vi "XYZ Stage Loop.vi"(6 "Used functions":bool, 8 "error in":errorcluster, 9 "Configuration":T1={"Parameter Analizer"={"Parameter Analyzer VISA Session"="COM1", "Sweeping Time Parameters"={"Integration Time"=0, "Short Integration Time (s)"=1.0, "Long Integration Time (s)"=0.0, "Wait Time Parameter"=1.0}, "Acquisition Mode"=enum."Sweeping Mode", "Status Polling Time (ms)"=0, "Comment"="Test VI", "SMU 1 - Sweeping"={"Start / Offset"=0.0, "Stop / Ratio"=1.0, "Step \n(linear only)"=0.01, "Compliance"=0.1, "Power \nCompliance"=0.0, "Mode"=0, "Function"=0, "Sweep Mode"=FALSE}, "SMU 2 - Sweeping"={"Start / Offset"=0.0, "Stop / Ratio"=1.0, "Step \n(linear only)"=0.01, "Compliance"=0.1, "Power \nCompliance"=0.0, "Mode"=0, "Function"=0, "Sweep Mode"=FALSE}, "SMU 3 - Sweeping"={"Start / Offset"=0.0, "Stop / Ratio"=1.0, "Step \n(linear only)"=0.01, "Compliance"=0.1, "Power \nCompliance"=0.0, "Mode"=0, "Function"=0, "Sweep Mode"=FALSE}, "SMU 4 - Sweeping"={"Start / Offset"=0.0, "Stop / Ratio"=1.0, "Step \n(linear only)"=0.01, "Compliance"=0.1, "Power \nCompliance"=0.0, "Mode"=0, "Function"=0, "Sweep Mode"=FALSE}, "Sweep Spacing"=0, "Range"=0, "SMU1 - Sampling"={"Source"=10.0, "Compliance"=1e-05, "Mode"=0, "Function"=FALSE}, "SMU2 - Sampling"={"Source"=1.0, "Compliance"=1.0, "Mode"=0, "Function"=FALSE}, "SMU3 - Sampling"={"Source"=10.0, "Compliance"=1e-05, "Mode"=0, "Function"=FALSE}, "SMU4 - Sampling"={"Source"=0.1, "Compliance"=60.0, "Mode"=10, "Function"=FALSE}, "Sampling Time Parameters"={"Initial Interval (s)"=0.1, "Number of Samples"=60, "Total Sampling Time (s)"=10.0, "Hold Time (s)"=0.0, "Sampling Mode"=0, "Sampling Time"=0}, "Stop Condition"={"Enable Delay (s)"=0.0, "Name"="", "Threshold"=0.0, "num. of events"=1, "Event"=0, "Stop Condition Enable"=FALSE}}, "Switching Matrix"={"Switching Matrix VISA Session"="GPIB0::18::INSTR", "Connections"=[{"Connections"=[FALSE, FALSE, FALSE, FALSE, FALSE, FALSE, FALSE, FALSE, FALSE, FALSE, FALSE, FALSE], "Connection Type"=enum."Disconnected"}, {"Connections"=[FALSE, FALSE, FALSE, FALSE, FALSE, FALSE, FALSE, FALSE, FALSE, FALSE, FALSE, FALSE], "Connection Type"=enum."Disconnected"}, {"Connections"=[FALSE, FALSE, FALSE, FALSE, FALSE, FALSE, FALSE, FALSE, FALSE, FALSE, FALSE, FALSE], "Connection Type"=enum."Disconnected"}, {"Connections"=[FALSE, FALSE, FALSE, FALSE, FALSE, FALSE, FALSE, FALSE, FALSE, FALSE, FALSE, FALSE], "Connection Type"=enum."Disconnected"}, {"Connections"=[FALSE, FALSE, FALSE, FALSE, FALSE, FALSE, FALSE, FALSE, FALSE, FALSE, FALSE, FALSE], "Connection Type"=enum."Disconnected"}, {"Connections"=[FALSE, FALSE, FALSE, FALSE, FALSE, FALSE, FALSE, FALSE, FALSE, FALSE, FALSE, FALSE], "Connection Type"=enum."Disconnected"}, {"Connections"=[FALSE, FALSE, FALSE, FALSE, FALSE, FALSE, FALSE, FALSE, FALSE, FALSE, FALSE, FALSE], "Connection Type"=enum."Disconnected"}, {"Connections"=[FALSE, FALSE, FALSE, FALSE, FALSE, FALSE, FALSE, FALSE, FALSE, FALSE, FALSE, FALSE], "Connection Type"=enum."Disconnected"}]}, "Stress Control"={"Stress Control VISA Session"="StrainMotor", "Axis"=0, "Motion"=0, "Destination (°)"=0.0, "Speed (°/s)"=4.0, "Position (°)"=25.0}, "Optical Spectrometer"={"Laser Settings"={"Laser Wavelength"=enum."365 nm", "Neutral Density Filter"=enum."100%"}, "Spectrometer Settings"={"Confocal Hole Size (µm)"=0.0, "Grating"=2, "Detector"=enum."InGaAs Array"}, "Acquisition Settings"={"Acquisition Mode"=enum."Multi-Window", "Spectal Position (nm)"=632.0, "From (nm)"=735.0, "To (nm)"=0.0, "Integration Time (s)"=0.0, "Number of Accumulations"=3, "AutoScanning"=FALSE, "Spike Removal"=FALSE}, "Path"=path "C:/07 - Prizes and Awards/Marie Curie Prize/Reply Editors Final NCOMMS(10).docx"}, "Switches & Mirrors"={"Relay VISA Session"="COM1", "Switches"={"Laser"=FALSE, "Video"=FALSE}, "Delays (ms)"={"Laser"=500, "Video"=1500}}, "Camera"={"Settings"={"Pixel clock"=20, "Frame rate"=30.0, "Exposure time"=33.21525, "Master Gain"=0, "Red Gain"=0, "Green Gain"=0, "Blue Gain"=0, "Auto Gain"=FALSE, "White-balance"=FALSE, "Color Correction"=FALSE}}, "XYZ Stage"={"Connection Settings"={"Tango VISA"="", "Baudrate"=57600, "Show Protocol?"=FALSE}, "Manual Control"={"North"=FALSE, "South"=FALSE, "West"=FALSE, "East"=FALSE, "Up"=FALSE, "Down"=FALSE, "Stop"=FALSE, "XY Step"=0.0, "Z step"=0.0}, "Coordinate Control"={"Motion Mode"=enum."Absolute", "Destination [mm]"=[]}}, "AutoFocus"={"Matching Criteria"={"Minimum Score"=700.0, "Color Score Weight"=700.0, "Minimum Contrast"=50, "Match Mode"=0, "Match Feature Mode"=0, "Subpixel Accuracy"=TRUE, "Color Sensitivity"=1, "Search Strategy"=1}, "Z Scan Parameters"={"Z Range"=1380.0, "Resolution"=5000.0, "Initial Direction"=enum."Up", "Focus Threshold"=0.1, "Ascent Constant"=0.1}, "Displacement"=0.0, "Transformation Matrix"=[]}, "Sava Data"={"Workspace Info"={"Device Name"="ProberHead_Tst_C29K3_7(2)", "Device Info"="ProberHead_Tst_C29", "Path"=path "C:/Users/gio/Desktop/ProbeHeadTest"}, "Instrument Configuration"={"Instrument"=enum."Unknown Instrument", "Configuration"="Test Configuration"}, "Stress Motor Position"=0.0, "Electrical Measurement"={"Sequence"=[], "V1"=[], "V2"=[], "V3"=[], "V4"=[], "I1"=[], "I2"=[], "I3"=[], "I4"=[]}, "Optical Spectrum"={"Intensity"=[], "Wavelength"=[], "Energy"=[], "Raman Shift"=[], "Detector Temperature"=0.0}}, "PlotData"={"Sliders"={"Strain Sequence"=0, "Instrument Sequence"=0}, "Measurement"={"Which Instrument?"=enum."No Plot", "Electrical Measurement"={"Sequence"=[], "V1"=[], "V2"=[], "V3"=[], "V4"=[], "I1"=[], "I2"=[], "I3"=[], "I4"=[]}, "Measurement Mode"=enum."Sweeping Mode", "Optical Spectrum"={"Intensity"=[], "Wavelength"=[], "Energy"=[], "Raman Shift"=[], "Detector Temperature"=0.0}}, "Instrument Steps"=[], "Strain Points"=[]}, "Instrument Sequence"={"Caller VI"=enum."User"}, "Strain Measurement"={"Stress Sequence "={"Max Motor Position"=1380.0, "# Intermediate Points"=5000, "Initial Direction"=enum."Tension"}, "Track?"=FALSE}} {"AutoFocus"."Displacement" scale=1.0..1000.0; "AutoFocus"."Z Scan Parameters"."Focus Threshold" min=0.0 max=1000.0 step=1.0 format="%#_2f"; "AutoFocus"."Z Scan Parameters"."Ascent Constant" min=0.0 max=1000.0 step=1.0 format="%#_2f"; "AutoFocus"."Z Scan Parameters"."Resolution" min=0.0 max=1.0 step=0.01 format="%_2g"; "AutoFocus"."Z Scan Parameters"."Z Range" format="%_3g"; "AutoFocus"."Matching Criteria"."Match Mode" items=["Shift Invariant", "Rotation Invariant"]; "AutoFocus"."Matching Criteria"."Match Feature Mode" items=["Color and Shape", "Color", "Shape"]; "AutoFocus"."Matching Criteria"."Color Sensitivity" items=["Low Sensitivity", "Medium Sensitivity", "High Sensitivity"]; "AutoFocus"."Matching Criteria"."Search Strategy" items=["Conservative", "Balance", "Aggressive", "Very Aggressive"]; "XYZ Stage"."Manual Control"."Z step" scale=0.1..10.0; "XYZ Stage"."Manual Control"."XY Step" scale=0.1..1000.0; "Camera"."Settings"."Blue Gain" min=0 max=100 scale=0.0..100.0; "Camera"."Settings"."Green Gain" min=0 max=100 scale=0.0..100.0; "Camera"."Settings"."Red Gain" min=0 max=100 scale=0.0..100.0; "Camera"."Settings"."Master Gain" min=0 max=100 scale=0.0..100.0; "Camera"."Settings"."Exposure time" min=0.101625 max=159.246375 step=0.101625 scale=0.101625..159.246375 scale format="%#.3g"; "Camera"."Settings"."Frame rate" min=2.7455631699174137 max=6.2675785993528725 step=0.000101625 scale=2.7455631699174137..6.2675785993528725 scale format="%^#_3g"; "Camera"."Settings"."Pixel clock" min=5 max=43 scale=5.0..43.0; "PlotData"."Sliders"."Instrument Sequence" scale=0.0..10.0; "PlotData"."Sliders"."Strain Sequence" scale=0.0..10.0; "Strain Measurement"."Stress Sequence"."# Intermediate Points" max=1390; "Parameter Analizer"."Stop Condition"."Event" items=["Value > Threshold", "Value < Threshold", "| Value | > | Threshold |", "| Value | < | Threshold |"]; "Parameter Analizer"."Stop Condition"."Threshold" format="%^.2e"; "Parameter Analizer"."Stop Condition"."Enable Delay (s)" format="%.1f"; "Parameter Analizer"."Sampling Time Parameters"."Sampling Time" items=["Auto (linear only)", "No Limit", "Set Limit"]; "Parameter Analizer"."Sampling Time Parameters"."Sampling Mode" items=["Linear", "Log10", "Log25", "Log50", "Thinned Out"]; "Parameter Analizer"."Sampling Time Parameters"."Hold Time (s)" format="%.4f"; "Parameter Analizer"."Sampling Time Parameters"."Total Sampling Time (s)" format="%.1f"; "Parameter Analizer"."Sampling Time Parameters"."Initial Interval (s)" format="%^.3e"; "Parameter Analizer"."SMU 4 - Sweeping"."Function" items=["Disabled", "Var 1", "Var 2", "Var 1'", "Constant"]; "Parameter Analizer"."SMU 4 - Sweeping"."Mode" items=["V", "I", "V pulse", "I  pulse", "Common"]; "Parameter Analizer"."SMU 4 - Sweeping"."Power \nCompliance" format="%^.2e"; "Parameter Analizer"."SMU 4 - Sweeping"."Compliance" format="%^.2e"; "Parameter Analizer"."SMU 4 - Sweeping"."Step \n(linear only)" format="%^.4e"; "Parameter Analizer"."SMU 4 - Sweeping"."Stop / Ratio" format="%^.4e"; "Parameter Analizer"."SMU 4 - Sweeping"."Start / Offset" format="%^.4e"; "Parameter Analizer"."SMU 3 - Sweeping"."Function" items=["Disabled", "Var 1", "Var 2", "Var 1'", "Constant"]; "Parameter Analizer"."SMU 3 - Sweeping"."Mode" items=["V", "I", "V pulse", "I  pulse", "Common"]; "Parameter Analizer"."SMU 3 - Sweeping"."Power \nCompliance" format="%^.2e"; "Parameter Analizer"."SMU 3 - Sweeping"."Compliance" format="%^.2e"; "Parameter Analizer"."SMU 3 - Sweeping"."Step \n(linear only)" format="%^.4e"; "Parameter Analizer"."SMU 3 - Sweeping"."Stop / Ratio" format="%^.4e"; "Parameter Analizer"."SMU 3 - Sweeping"."Start / Offset" format="%^.4e"; "Parameter Analizer"."SMU 2 - Sweeping"."Function" items=["Disabled", "Var 1", "Var 2", "Var 1'", "Constant"]; "Parameter Analizer"."SMU 2 - Sweeping"."Mode" items=["V", "I", "V pulse", "I  pulse", "Common"]; "Parameter Analizer"."SMU 2 - Sweeping"."Power \nCompliance" format="%^.2e"; "Parameter Analizer"."SMU 2 - Sweeping"."Compliance" format="%^.2e"; "Parameter Analizer"."SMU 2 - Sweeping"."Step \n(linear only)" format="%^.4e"; "Parameter Analizer"."SMU 2 - Sweeping"."Stop / Ratio" format="%^.4e"; "Parameter Analizer"."SMU 2 - Sweeping"."Start / Offset" format="%^.4e"; "Parameter Analizer"."SMU 1 - Sweeping"."Function" items=["Disabled", "Var 1", "Var 2", "Var 1'", "Constant"]; "Parameter Analizer"."SMU 1 - Sweeping"."Mode" items=["V", "I", "V pulse", "I  pulse", "Common"]; "Parameter Analizer"."SMU 1 - Sweeping"."Power \nCompliance" format="%^.2e"; "Parameter Analizer"."SMU 1 - Sweeping"."Compliance" format="%^.2e"; "Parameter Analizer"."SMU 1 - Sweeping"."Step \n(linear only)" format="%^.4e"; "Parameter Analizer"."SMU 1 - Sweeping"."Stop / Ratio" format="%^.4e"; "Parameter Analizer"."SMU 1 - Sweeping"."Start / Offset" format="%^.4e"; "Parameter Analizer"."Sweeping Time Parameters"."Long Integration Time (s)" scale=0.02..2.0; "Parameter Analizer"."Sweeping Time Parameters"."Short Integration Time (s)" scale=8e-05..0.00192; "Parameter Analizer"."Sweeping Time Parameters"."Integration Time" items=["Short", "Long"]; "Parameter Analizer"."Sweeping Time Parameters"."Wait Time Parameter" format="%.1f"; "Parameter Analizer"."SMU4 - Sampling"."Mode" items=["V", "I", "Common"]; "Parameter Analizer"."SMU4 - Sampling"."Compliance" format="%^.2e"; "Parameter Analizer"."SMU4 - Sampling"."Source" format="%^.3e"; "Parameter Analizer"."SMU3 - Sampling"."Mode" items=["V", "I", "Common"]; "Parameter Analizer"."SMU3 - Sampling"."Compliance" format="%^.2e"; "Parameter Analizer"."SMU3 - Sampling"."Source" format="%^.3e"; "Parameter Analizer"."SMU2 - Sampling"."Mode" items=["V", "I", "Common"]; "Parameter Analizer"."SMU2 - Sampling"."Compliance" format="%^.2e"; "Parameter Analizer"."SMU2 - Sampling"."Source" format="%^.3e"; "Parameter Analizer"."SMU1 - Sampling"."Mode" items=["V", "I", "Common"]; "Parameter Analizer"."SMU1 - Sampling"."Compliance" format="%^.2e"; "Parameter Analizer"."SMU1 - Sampling"."Source" format="%^.3e"; "Parameter Analizer"."Range" items=["auto", "fixed", "limited"]; "Parameter Analizer"."Sweep Spacing" items=["linear", "log 10", "log 25", "log 50"]; "Stress Control"."Axis" min=1 max=3; "Stress Control"."Position (°)" format="%.6g"; "Stress Control"."Speed (°/s)" min=0.0 max=4.0 format="%.6f"; "Stress Control"."Destination (°)" min=-2000000000.0 max=2000000000.0 format="%.6f"; "Stress Control"."Motion" items=["Absolute", "Relative"]; "Optical Spectrometer"."Spectrometer Settings"."Grating" items=["1800 l/mm", "150 l/mm"]}, 10 "Message Queues out":T57, 11 "Notifiers":T44) -> (0 "error out":errorcluster)   [LabVIEW 2014]
uses:
  support/Message Queue/All Message Queues.ctl
  support/Message Queue/Message Cluster.ctl
  support/Notifiers/Notifiers.ctl
  support/Message Handler Loop Notifiers.ctl
  Hardware Control/Parameter Analyzer/Parameter Analyzer Notifiers.ctl
  Hardware Control/Switching Matrix/Switching Matrix Notifiers.ctl
  Hardware Control/Stress Control/StressControl Notifiers.ctl
  Hardware Control/Spectrometer/Spectrometer Notifiers.ctl
  Hardware Control/Switches and Mirrors/SwitchesMirrors Notifiers.ctl
  Hardware Control/Camera/Camera Notifiers.ctl
  Hardware Control/XYZ Stage/XYZ Notifications.ctl
  Hardware Control/Autofocus/Autofocus Notifiers.ctl
  Measurements/Optoelectronic Measurement/Optoelectronic Notifiers.ctl
  Measurements/Save Data/SaveData Notifiers.ctl
  Measurements/Instrument Sequence/Instrument Sequence Notifiers.ctl
  support/Configuration/Configuration.ctl
  Hardware Control/Parameter Analyzer/Parameter Analyzer Config.ctl
  Hardware Control/Parameter Analyzer/Parameter Analyzer Integration Parameters.ctl
  Hardware Control/Parameter Analyzer/Parameter Analyzer SMU Sweeping.ctl
  Hardware Control/Parameter Analyzer/Parameter Analyzer Sweep Spacing.ctl
  Hardware Control/Parameter Analyzer/Parameter Analyzer SMU Range.ctl
  Hardware Control/Parameter Analyzer/Parameter Analyzer SMU Sampling.ctl
  Hardware Control/Parameter Analyzer/Parameter Analyzer Sampling Parameters.ctl
  Hardware Control/Parameter Analyzer/Parameter Analyzer Stop Sampling Conditions.ctl
  Hardware Control/Switching Matrix/Switching Matrix Config.ctl
  Hardware Control/Stress Control/StressControl Config.ctl
  Hardware Control/Spectrometer/Spectrometer Config.ctl
  Hardware Control/Spectrometer/Laser Settings.ctl
  Hardware Control/Spectrometer/Laser.ctl
  Hardware Control/Spectrometer/Filter.ctl
  Hardware Control/Spectrometer/Grating Detector Settings.ctl
  Hardware Control/Spectrometer/Grating.ctl
  Hardware Control/Spectrometer/Detector.ctl
  Hardware Control/Spectrometer/Acquisition Settings.ctl
  Hardware Control/Switches and Mirrors/SwitchesMirrors Config.ctl
  Hardware Control/Switches and Mirrors/SwitchesMirrors Status.ctl
  Hardware Control/Camera/Camera Config.ctl
  Hardware Control/Camera/Camera Settings.ctl
  Hardware Control/XYZ Stage/XYZ Config.ctl
  Hardware Control/XYZ Stage/XYZ Connection Settings.ctl
  Hardware Control/XYZ Stage/XYZ Stage Control.ctl
  Hardware Control/XYZ Stage/XYZ Coordinate Control.ctl
  Hardware Control/Autofocus/AutoFocus Config.ctl
  Hardware Control/Autofocus/ZScan.ctl
  <vilib>/Analysis/Matrix/Datatypes/RealMatrix.ctl
  Measurements/Save Data/SaveData Config.ctl
  Measurements/Save Data/SaveData Workspace Info.ctl
  Measurements/Save Data/SaveData Instrument Configuration.ctl
  Measurements/Instrument Sequence/Instrument List.ctl
  Hardware Control/Spectrometer/Spectral Data.ctl
  Measurements/Plot Data/PlotData Config.ctl
  Measurements/Plot Data/Measurement.ctl
  Measurements/Plot Data/WhichInstrument.ctl
  Hardware Control/Parameter Analyzer/Electrical Data.ctl
  Measurements/Instrument Sequence/Instrument Steps.ctl
  Measurements/Instrument Sequence/Action.ctl
  Measurements/Instrument Sequence/Instrument Sequence Config.ctl
  Measurements/Strain Measurement/Strain Measurement Config.ctl
  Hardware Control/XYZ Stage/XYZ Function.ctl
  support/Message Queue/Message Queue.lvlib
  <vilib>/Analysis/Matrix/NI_Matrix.lvlib
panel:
  # "LICENSED MATERIALS – PROPERTY OF IBM\nCopyright IBM Corp. 2016,\nALL RIGHTS RESERVED"
  # "XY"
  # "Z"
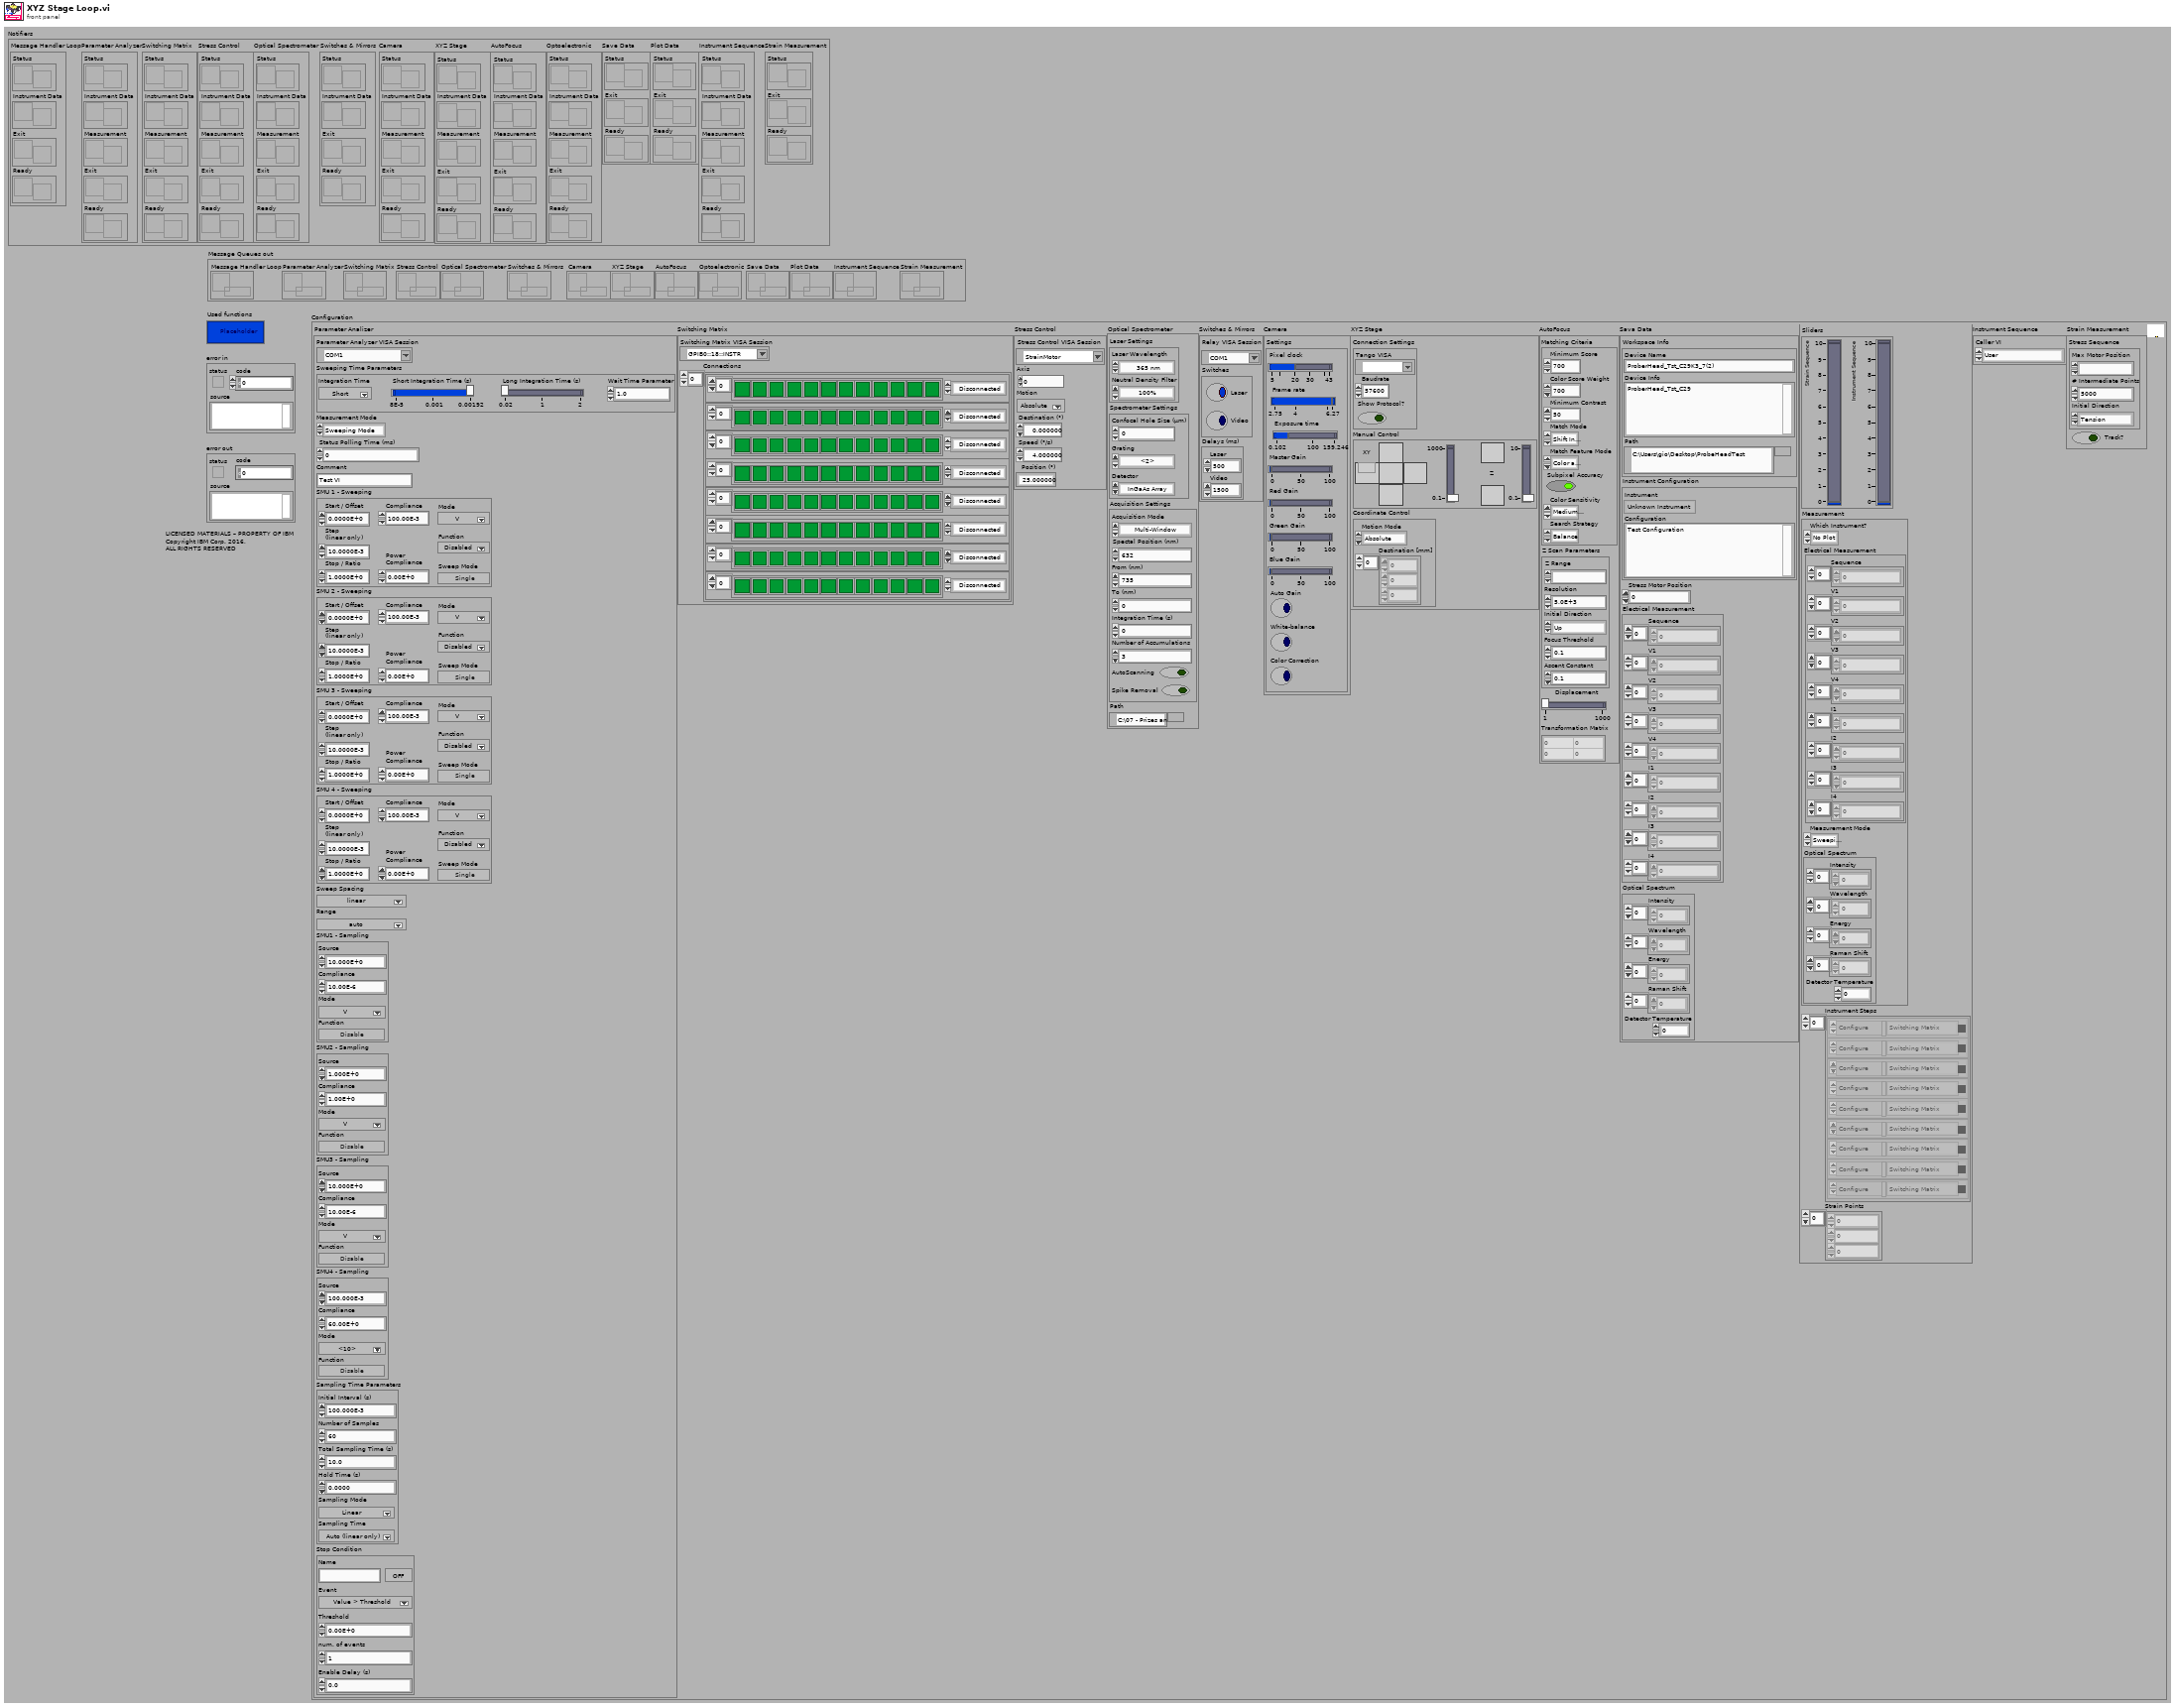
[diagram p1: front panel]
types:
  T1 = typedef "Configuration.ctl" = cluster{"Parameter Analizer":T2, "Switching Matrix":T10, "Stress Control":T11, "Optical Spectrometer":T12, "Switches & Mirrors":T20, "Camera":T22, "XYZ Stage":T24, "AutoFocus":T28, "Sava Data":T31, "PlotData":T36, "Instrument Sequence":T42, "Strain Measurement":T43}
  T2 = typedef "Parameter Analyzer Config.ctl" = cluster{"Parameter Analyzer VISA Session":refnum<visa-resource-name>, "Sweeping Time Parameters":T3, "Acquisition Mode":enum32{"Sweeping Mode", "Sampling Mode"}, "Status Polling Time (ms)":u32, "Comment":string, "SMU 1 - Sweeping":T4, "SMU 2 - Sweeping":T4, "SMU 3 - Sweeping":T4, "SMU 4 - Sweeping":T4, "Sweep Spacing":T5, "Range":T6, "SMU1 - Sampling":T7, "SMU2 - Sampling":T7, "SMU3 - Sampling":T7, "SMU4 - Sampling":T7, "Sampling Time Parameters":T8, "Stop Condition":T9}
  T3 = typedef "Parameter Analyzer Integration Parameters.ctl" = cluster{"Integration Time":u32, "Short Integration Time (s)":dbl, "Long Integration Time (s)":dbl, "Wait Time Parameter":dbl}
  T4 = typedef "Parameter Analyzer SMU Sweeping.ctl" = cluster{"Start / Offset":dbl, "Stop / Ratio":dbl, "Step \n(linear only)":dbl, "Compliance":dbl, "Power \nCompliance":dbl, "Mode":u32, "Function":i32, "Sweep Mode":bool}
  T5 = typedef "Parameter Analyzer Sweep Spacing.ctl" = u16
  T6 = typedef "Parameter Analyzer SMU Range.ctl" = u16
  T7 = typedef "Parameter Analyzer SMU Sampling.ctl" = cluster{"Source":dbl, "Compliance":dbl, "Mode":u32, "Function":bool}
  T8 = typedef "Parameter Analyzer Sampling Parameters.ctl" = cluster{"Initial Interval (s)":dbl, "Number of Samples":i32, "Total Sampling Time (s)":dbl, "Hold Time (s)":dbl, "Sampling Mode":i32, "Sampling Time":i32}
  T9 = typedef "Parameter Analyzer Stop Sampling Conditions.ctl" = cluster{"Enable Delay (s)":dbl, "Name":string, "Threshold":dbl, "num. of events":i32, "Event":i32, "Stop Condition Enable":bool}
  T10 = typedef "Switching Matrix Config.ctl" = cluster{"Switching Matrix VISA Session":refnum<visa-resource-name>, "Connections":cluster{"Connections":bool[], "Connection Type":enum16{"Disconnected", "Make - Break", "Break - Make"}}[]}
  T11 = typedef "StressControl Config.ctl" = cluster{"Stress Control VISA Session":refnum<visa-resource-name>, "Axis":i32, "Motion":u16, "Destination (°)":dbl, "Speed (°/s)":dbl, "Position (°)":dbl}
  T12 = typedef "Spectrometer Config.ctl" = cluster{"Laser Settings":T13, "Spectrometer Settings":T16, "Acquisition Settings":T19, "Path":path}
  T13 = typedef "Laser Settings.ctl" = cluster{"Laser Wavelength":T14, "Neutral Density Filter":T15}
  T14 = typedef "Laser.ctl" = enum16{"633 nm", "784 nm", "532 nm", "365 nm"}
  T15 = typedef "Filter.ctl" = enum16{"100%", "50%", "25%", "10%", "1%", "0.1%", "0.01%"}
  T16 = typedef "Grating Detector Settings.ctl" = cluster{"Confocal Hole Size (µm)":dbl, "Grating":T17, "Detector":T18}
  T17 = typedef "Grating.ctl" = u16
  T18 = typedef "Detector.ctl" = enum16{"InGaAs Array", "Silicon CCD"}
  T19 = typedef "Acquisition Settings.ctl" = cluster{"Acquisition Mode":enum16{"Single Window", "Multi-Window"}, "Spectal Position (nm)":dbl, "From (nm)":dbl, "To (nm)":dbl, "Integration Time (s)":dbl, "Number of Accumulations":i32, "AutoScanning":bool, "Spike Removal":bool}
  T20 = typedef "SwitchesMirrors Config.ctl" = cluster{"Relay VISA Session":refnum<visa-resource-name>, "Switches":T21, "Delays (ms)":cluster{"Laser":u32, "Video":u32}}
  T21 = typedef "SwitchesMirrors Status.ctl" = cluster{"Laser":bool, "Video":bool}
  T22 = typedef "Camera Config.ctl" = cluster{"Settings":T23}
  T23 = typedef "Camera Settings.ctl" = cluster{"Pixel clock":i32, "Frame rate":dbl, "Exposure time":dbl, "Master Gain":i32, "Red Gain":i32, "Green Gain":i32, "Blue Gain":i32, "Auto Gain":bool, "White-balance":bool, "Color Correction":bool}
  T24 = typedef "XYZ Config.ctl" = cluster{"Connection Settings":T25, "Manual Control":T26, "Coordinate Control":T27}
  T25 = typedef "XYZ Connection Settings.ctl" = cluster{"Tango VISA":refnum<visa-resource-name>, "Baudrate":i32, "Show Protocol?":bool}
  T26 = typedef "XYZ Stage Control.ctl" = cluster{"North":bool, "South":bool, "West":bool, "East":bool, "Up":bool, "Down":bool, "Stop":bool, "XY Step":dbl, "Z step":dbl}
  T27 = typedef "XYZ Coordinate Control.ctl" = cluster{"Motion Mode":enum16{"Absolute", "Relative"}, "Destination [mm]":dbl[]}
  T28 = typedef "AutoFocus Config.ctl" = cluster{"Matching Criteria":cluster{"Minimum Score":sgl, "Color Score Weight":sgl, "Minimum Contrast":i32, "Match Mode":u32, "Match Feature Mode":u32, "Subpixel Accuracy":bool, "Color Sensitivity":u32, "Search Strategy":u32}, "Z Scan Parameters":T29, "Displacement":dbl, "Transformation Matrix":T30}
  T29 = typedef "ZScan.ctl" = cluster{"Z Range":ext, "Resolution":dbl, "Initial Direction":enum16{"Up", "Down"}, "Focus Threshold":dbl, "Ascent Constant":dbl}
  T30 = typedef "NI_Matrix.lvlib/RealMatrix.ctl" = dbl[][]
  T31 = typedef "SaveData Config.ctl" = cluster{"Workspace Info":T32, "Instrument Configuration":T33, "Stress Motor Position":dbl, "Electrical Measurement":cluster{"Sequence":dbl[], "V1":dbl[], "V2":dbl[], "V3":dbl[], "V4":dbl[], "I1":dbl[], "I2":dbl[], "I3":dbl[], "I4":dbl[]}, "Optical Spectrum":T35}
  T32 = typedef "SaveData Workspace Info.ctl" = cluster{"Device Name":string, "Device Info":string, "Path":path}
  T33 = typedef "SaveData Instrument Configuration.ctl" = cluster{"Instrument":T34, "Configuration":string}
  T34 = typedef "Instrument List.ctl" = enum32{"Unknown Instrument", "Switching Matrix", "Parameter Analyzer", "Optical Spectrometer", "Optoelectronic", "Autofocus"}
  T35 = typedef "Spectral Data.ctl" = cluster{"Intensity":dbl[], "Wavelength":dbl[], "Energy":dbl[], "Raman Shift":dbl[], "Detector Temperature":dbl}
  T36 = typedef "PlotData Config.ctl" = cluster{"Sliders":cluster{"Strain Sequence":i32, "Instrument Sequence":i32}, "Measurement":T37, "Instrument Steps":T40, "Strain Points":dbl[]}
  T37 = typedef "Measurement.ctl" = cluster{"Which Instrument?":T38, "Electrical Measurement":T39, "Measurement Mode":enum16{"Sweeping Mode", "Sampling Mode"}, "Optical Spectrum":T35}
  T38 = typedef "WhichInstrument.ctl" = enum16{"No Plot", "Spectrometer", "Parameter Analyzer", "Optoelectronic"}
  T39 = typedef "Electrical Data.ctl" = cluster{"Sequence":dbl[], "V1":dbl[], "V2":dbl[], "V3":dbl[], "V4":dbl[], "I1":dbl[], "I2":dbl[], "I3":dbl[], "I4":dbl[]}
  T40 = typedef "Instrument Steps.ctl" = cluster{"Action":T41, "Configuration":variant, "Instrument":T34, "Status":enum8{"False", "True", "Mixed"}}[]
  T41 = typedef "Action.ctl" = enum32{"Configure", "Measure"}
  T42 = typedef "Instrument Sequence Config.ctl" = cluster{"Caller VI":enum16{"User", "Stress Measurement VI"}}
  T43 = typedef "Strain Measurement Config.ctl" = cluster{"Stress Sequence ":cluster{"Max Motor Position":ext, "# Intermediate Points":u32, "Initial Direction":enum16{"Tension", "Compression"}}, "Track?":bool}
  T44 = typedef "Notifiers.ctl" = cluster{"Message Handler Loop":T45, "Parameter Analyzer":T46, "Switching Matrix":T47, "Stress Control":T48, "Optical Spectrometer":T49, "Switches & Mirrors":T50, "Camera":T51, "XYZ Stage":T52, "AutoFocus":T53, "Optoelectronic":T54, "Save Data":T55, "Plot Data":T55, "Instrument Sequence":T56, "Strain Measurement":cluster{"Status":refnum<notifier>, "Exit":refnum<notifier>, "Ready":refnum<notifier>}}
  T45 = typedef "Message Handler Loop Notifiers.ctl" = cluster{"Status":refnum<notifier>, "Instrument Data":refnum<notifier>, "Exit":refnum<notifier>, "Ready":refnum<notifier>}
  T46 = typedef "Parameter Analyzer Notifiers.ctl" = cluster{"Status":refnum<notifier>, "Instrument Data":refnum<notifier>, "Measurement":refnum<notifier>, "Exit":refnum<notifier>, "Ready":refnum<notifier>}
  T47 = typedef "Switching Matrix Notifiers.ctl" = cluster{"Status":refnum<notifier>, "Instrument Data":refnum<notifier>, "Measurement":refnum<notifier>, "Exit":refnum<notifier>, "Ready":refnum<notifier>}
  T48 = typedef "StressControl Notifiers.ctl" = cluster{"Status":refnum<notifier>, "Instrument Data":refnum<notifier>, "Measurement":refnum<notifier>, "Exit":refnum<notifier>, "Ready":refnum<notifier>}
  T49 = typedef "Spectrometer Notifiers.ctl" = cluster{"Status":refnum<notifier>, "Instrument Data":refnum<notifier>, "Measurement":refnum<notifier>, "Exit":refnum<notifier>, "Ready":refnum<notifier>}
  T50 = typedef "SwitchesMirrors Notifiers.ctl" = cluster{"Status":refnum<notifier>, "Instrument Data":refnum<notifier>, "Exit":refnum<notifier>, "Ready":refnum<notifier>}
  T51 = typedef "Camera Notifiers.ctl" = cluster{"Status":refnum<notifier>, "Instrument Data":refnum<notifier>, "Measurement":refnum<notifier>, "Exit":refnum<notifier>, "Ready":refnum<notifier>}
  T52 = typedef "XYZ Notifications.ctl" = cluster{"Status":refnum<notifier>, "Instrument Data":refnum<notifier>, "Measurement":refnum<notifier>, "Exit":refnum<notifier>, "Ready":refnum<notifier>}
  T53 = typedef "Autofocus Notifiers.ctl" = cluster{"Status":refnum<notifier>, "Instrument Data":refnum<notifier>, "Measurement":refnum<notifier>, "Exit":refnum<notifier>, "Ready":refnum<notifier>}
  T54 = typedef "Optoelectronic Notifiers.ctl" = cluster{"Status":refnum<notifier>, "Instrument Data":refnum<notifier>, "Measurement":refnum<notifier>, "Exit":refnum<notifier>, "Ready":refnum<notifier>}
  T55 = typedef "SaveData Notifiers.ctl" = cluster{"Status":refnum<notifier>, "Exit":refnum<notifier>, "Ready":refnum<notifier>}
  T56 = typedef "Instrument Sequence Notifiers.ctl" = cluster{"Status":refnum<notifier>, "Instrument Data":refnum<notifier>, "Measurement":refnum<notifier>, "Exit":refnum<notifier>, "Ready":refnum<notifier>}
  T57 = typedef "Message Queue.lvlib/All Message Queues.ctl" = cluster{"Message Handler Loop":refnum<queue>, "Parameter Analyzer":refnum<queue>, "Switching Matrix":refnum<queue>, "Stress Control":refnum<queue>, "Optical Spectrometer":refnum<queue>, "Switches & Mirrors":refnum<queue>, "Camera":refnum<queue>, "XYZ Stage":refnum<queue>, "AutoFocus":refnum<queue>, "Optoelectronic":refnum<queue>, "Save Data":refnum<queue>, "Plot Data":refnum<queue>, "Instrument Sequence":refnum<queue>, "Strain Measurement":refnum<queue>}
  T58 = typedef "XYZ Data.ctl" = cluster{"Configuration":T24, "Refnums":T59, "Initialization":T60}
  T59 = typedef "XYZ Refnums.ctl" = cluster{"Instrument Status":refnum<vi>, "Position":refnum<vi>, "Manual Control":refnum<vi>, "Up":refnum<vi>, "Down":refnum<vi>, "North":refnum<vi>, "South":refnum<vi>, "East":refnum<vi>, "West":refnum<vi>, "Stop":refnum<vi>, "Limits":refnum<vi>}
  T60 = typedef "XYZ Initialization.ctl" = cluster{"Update Visa Session":bool, "Set To Default":bool, "Get Status":bool, "Update Refnums":bool}
  T61 = typedef "XYZ Function.ctl" = enum16{"Connect", "Initialize", "Calibrate", "Meaure Range", "Limits", "Center", "Set Zero", "Velocity", "Manual Control", "Coordinate Move", "Move with Backlash Compensation", "Meander", "Sequence", "Analog Output", "Send Command", "Show Protocol", "Get Status", "Disconnect", "Update Refnums"}
  T62 = cluster{"Connected?":bool, "LSID":i32, "Position":dbl[], "Number of Axes":u8}
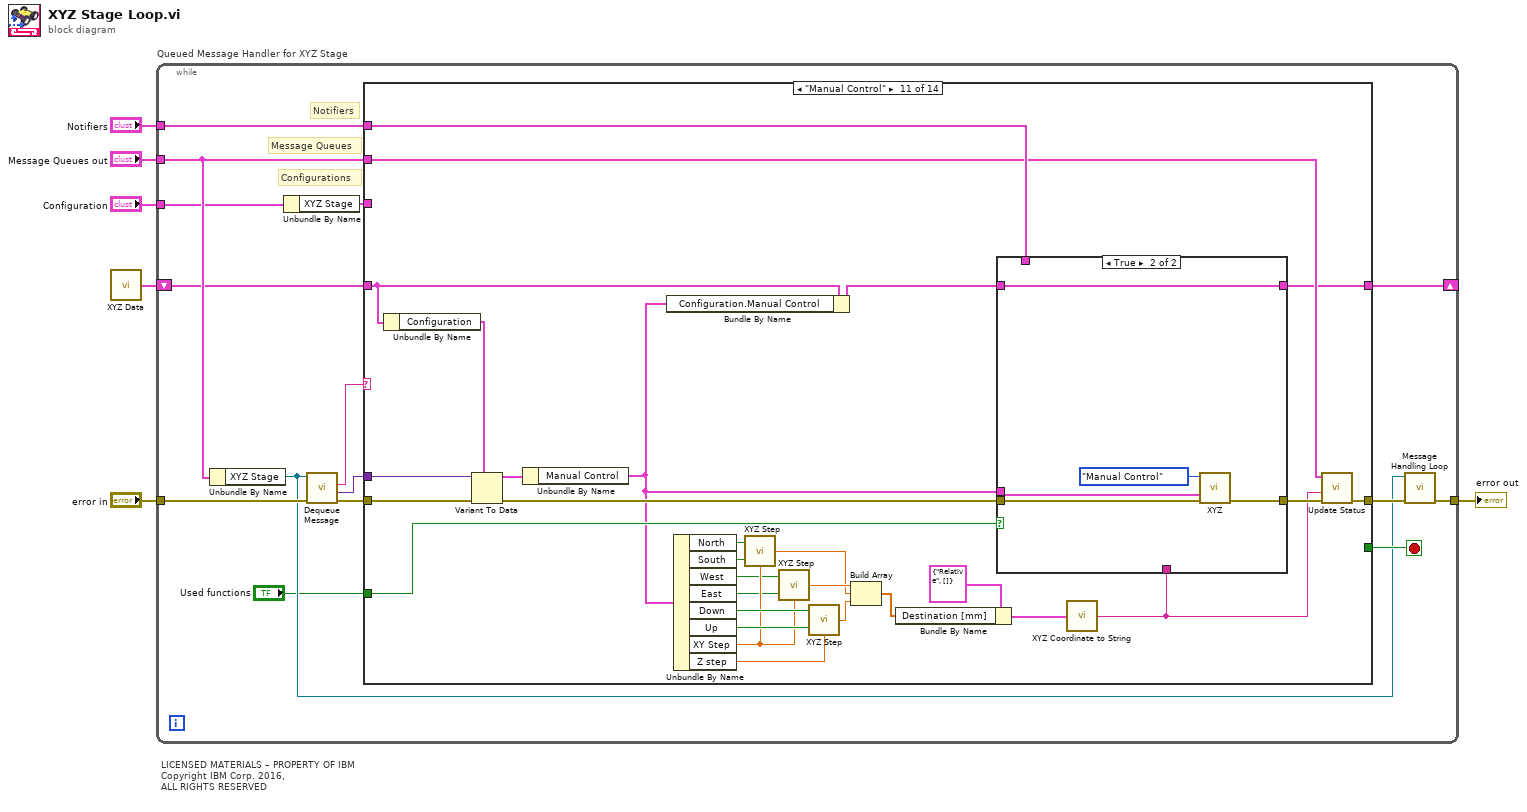
[diagram p0: block diagram]
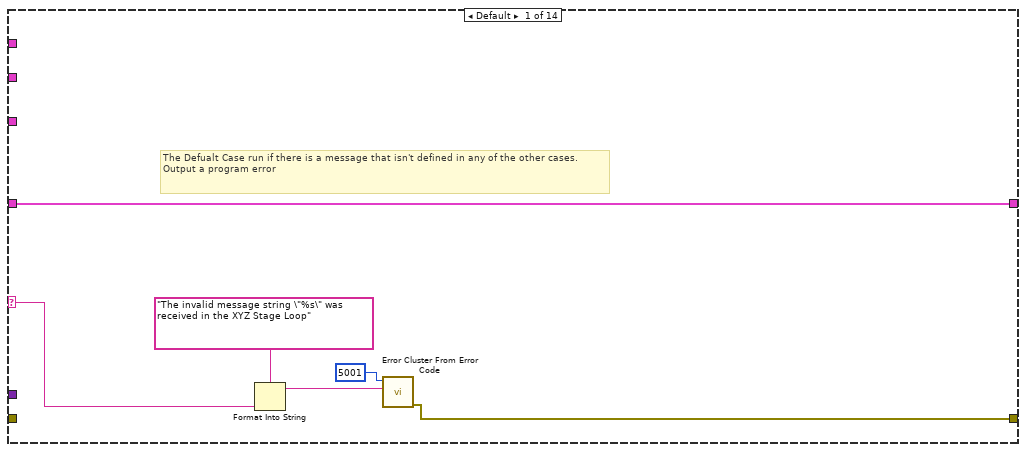
[diagram p2: hidden frame]
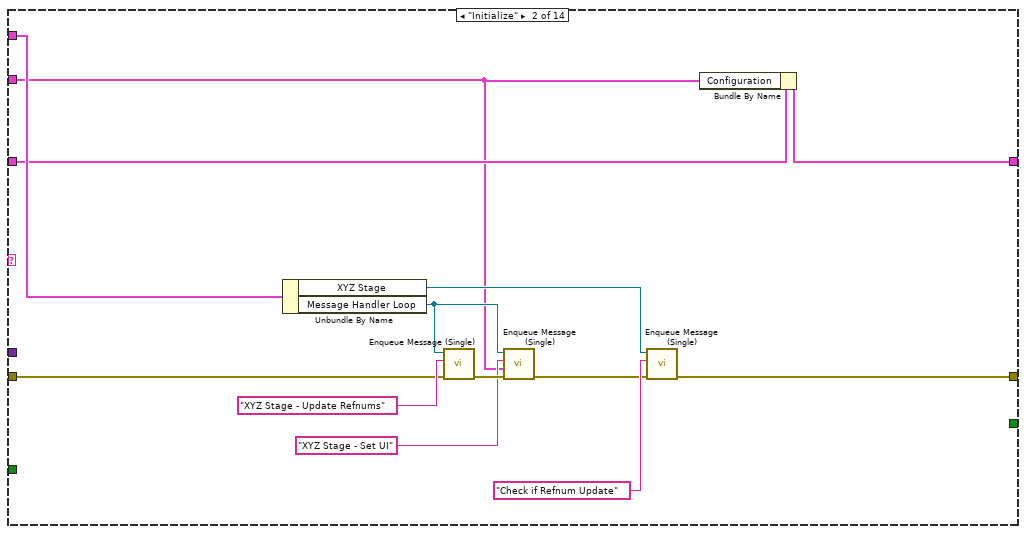
[diagram p3: hidden frame]
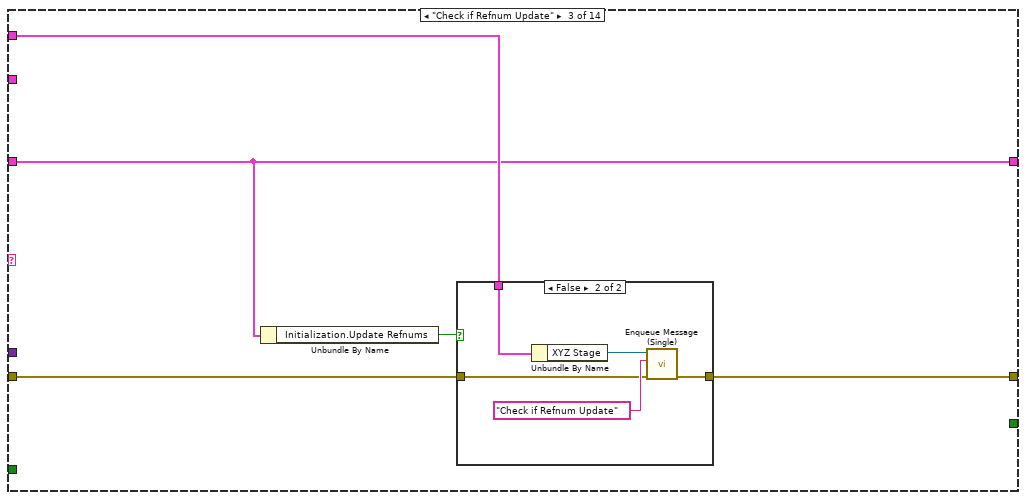
[diagram p4: hidden frame]
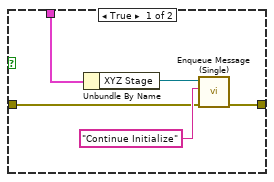
[diagram p5: hidden frame]
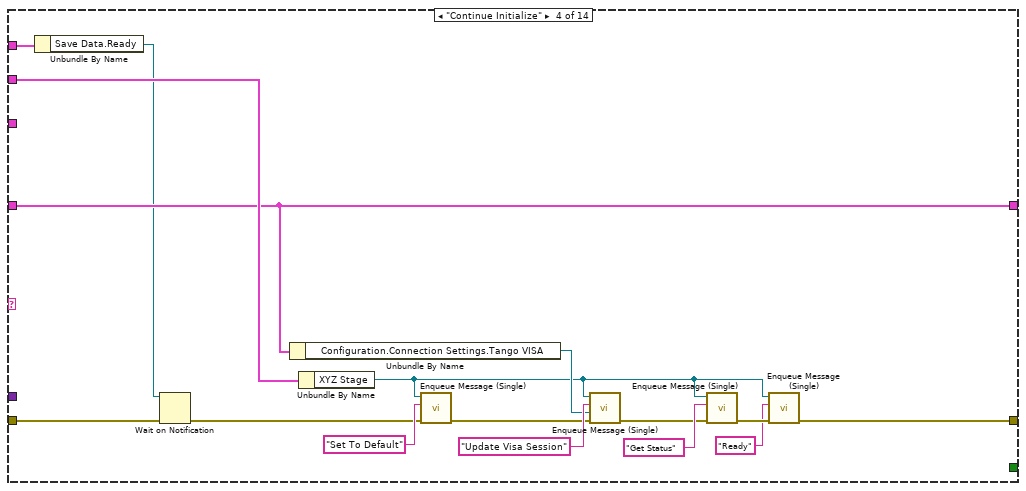
[diagram p6: hidden frame]
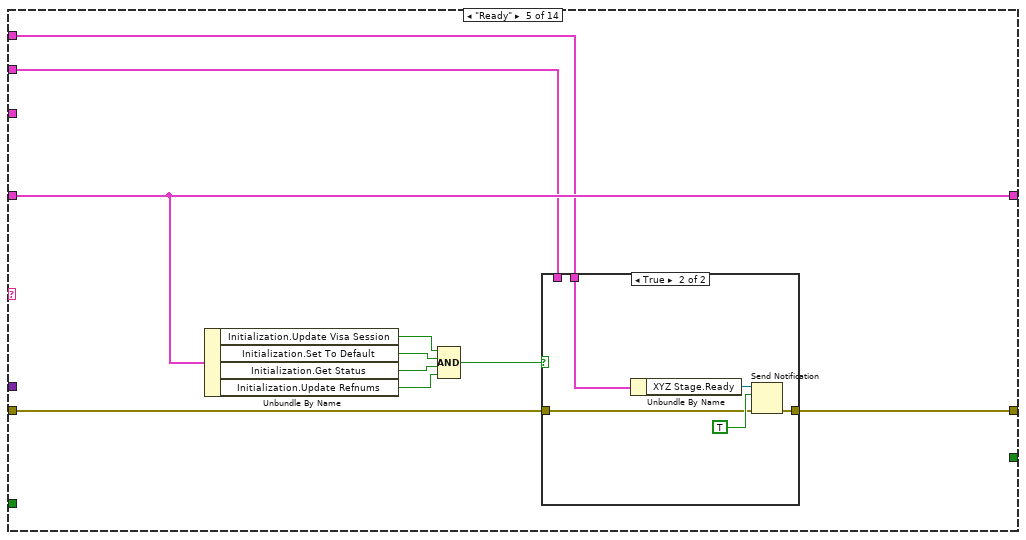
[diagram p7: hidden frame]
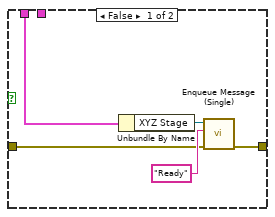
[diagram p8: hidden frame]
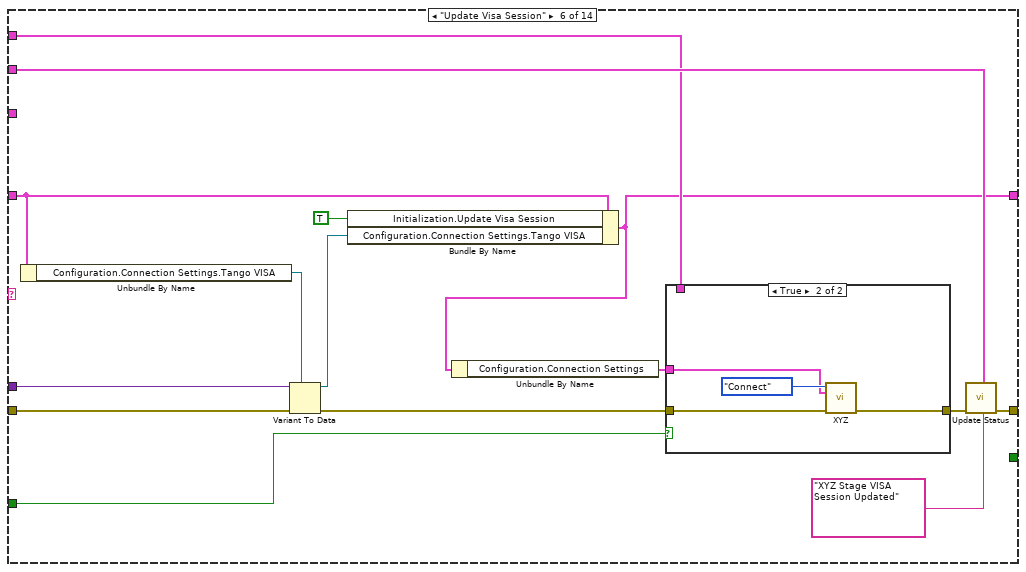
[diagram p9: hidden frame]
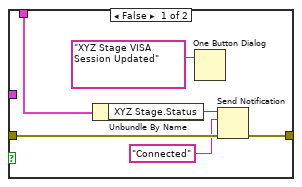
[diagram p10: hidden frame]
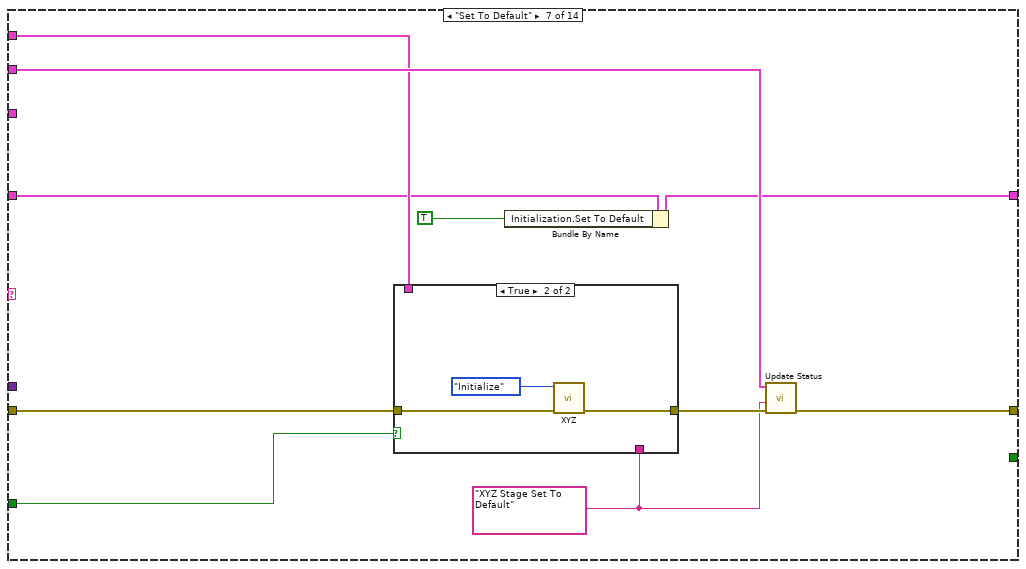
[diagram p11: hidden frame]
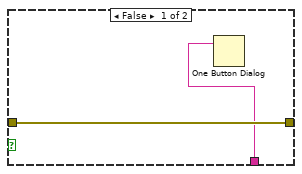
[diagram p12: hidden frame]
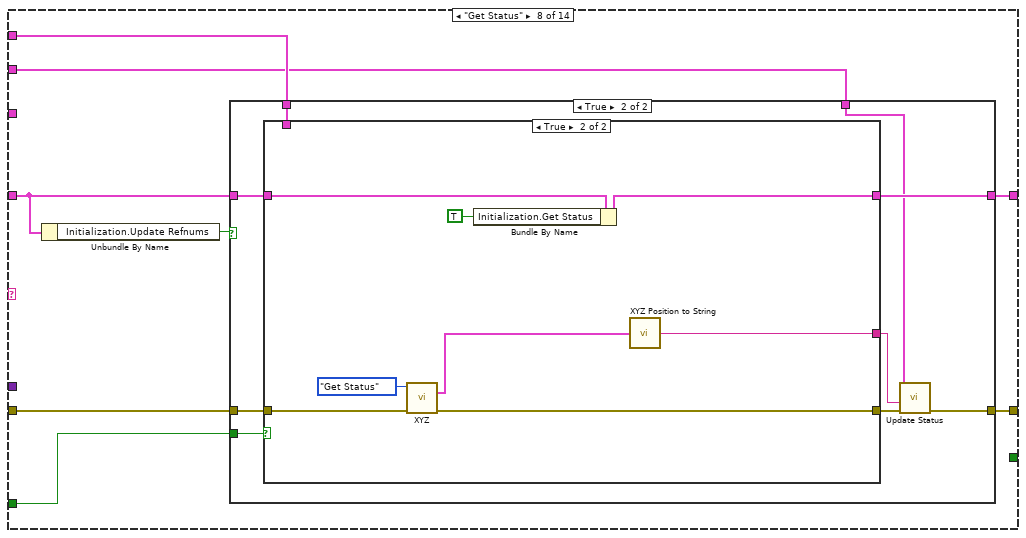
[diagram p13: hidden frame]
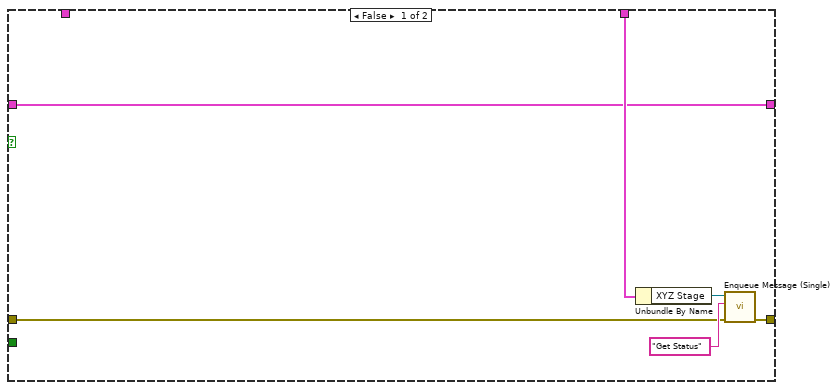
[diagram p14: hidden frame]
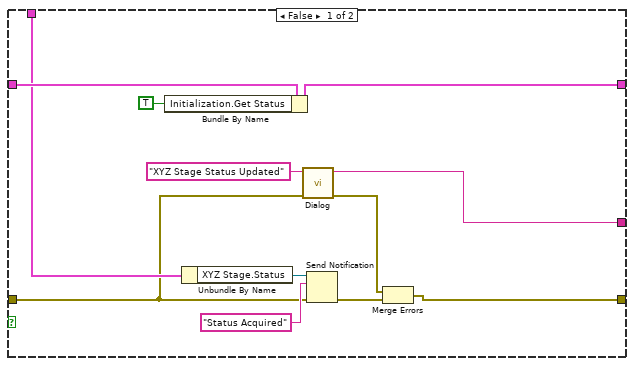
[diagram p15: hidden frame]
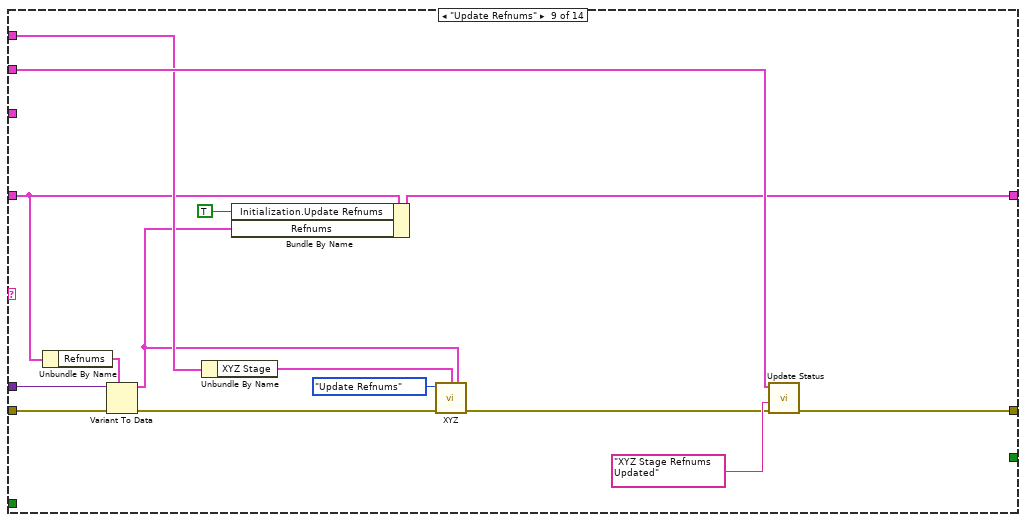
[diagram p16: hidden frame]
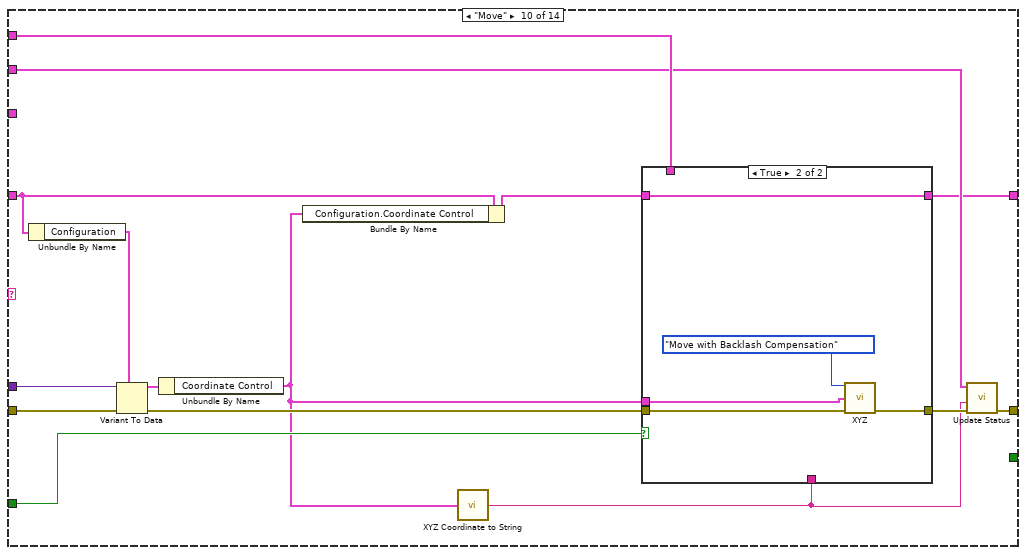
[diagram p17: hidden frame]
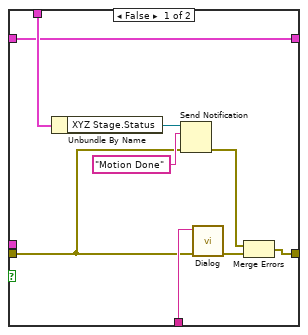
[diagram p18: hidden frame]
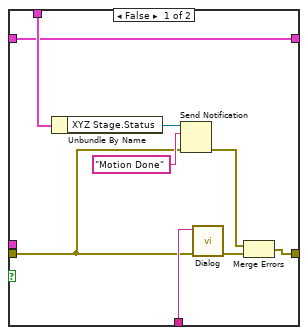
[diagram p19: hidden frame]
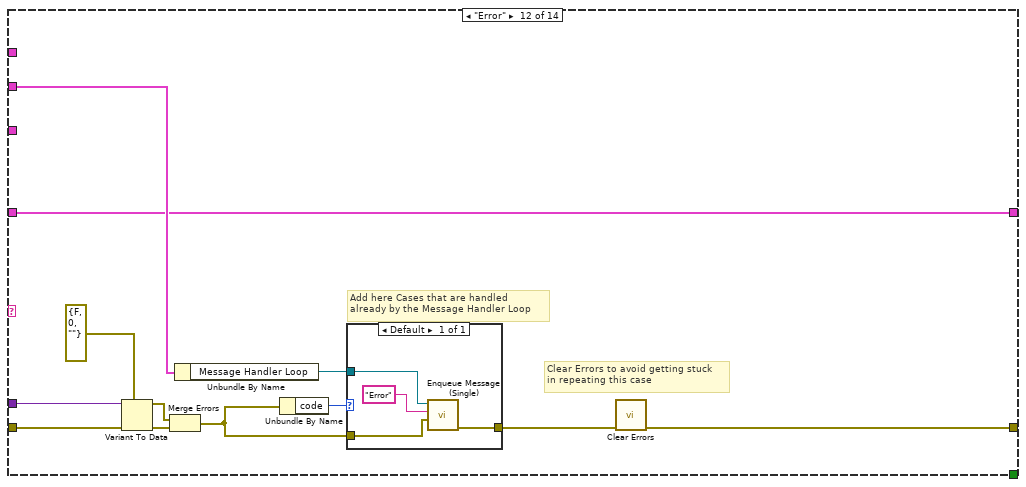
[diagram p20: hidden frame]
diagram:
  # "LICENSED MATERIALS – PROPERTY OF IBM\nCopyright IBM Corp. 2016,\nALL RIGHTS RESERVED"
  n1 = call "XYZ Data.vi"() -> ("XYZ Stage Data"=w1:T58)
  n2 = while "Queued Message Handler for XYZ Stage" {
    tunnel: "error in" -> [w21]
    tunnel: [w13] -> w2
    tunnel: "Message Queues out" -> [w17]
    tunnel: "Notifiers" -> [w16]
    tunnel: "Configuration" -> [w11]
    shift-right: [w7] -> _
    shift-left: w1 -> [w8]
    stop <- w15 stop-if-true
    # "Configurations"
    # "Notifiers"
    # "Message Queues"
    n3 = Unbundle By Name(w17) -> ("XYZ Stage"=w12:refnum<queue>)
    n4 = Unbundle By Name(w11) -> ("XYZ Stage"=w10:T24)
    n5 = call "Dequeue Message.vi"("error in (no error)"=w21, "Message Queue"=w12) -> ("error out"=w20:errorcluster, "Message Data"=w18:variant, "Message"=w19:string)  [unwired: 7 out]
    n6 = case shown="\"Manual Control\"" w19 {
      selector: w19 -> [w24 _ _ _ _ _ _ _ _ _ _ _ _ _]
      tunnel: w20 -> [_ w28 w43 w57 w75 w104 w118 w134 w187 w201 w244 w269 w287 w303]
      tunnel: [w23 w29 w44 w68 w73 w102 w125 w132 w186 w199 w242 w264 w277 w302] -> w14
      tunnel: w18 -> [_ _ _ _ _ w106 _ _ w188 w203 w246 w262 _ _]
      tunnel: w17 -> [_ w40 w45 w71 w74 w101 w124 w135 w184 w195 w238 w270 w289 _]
      tunnel: w16 -> [_ _ _ w58 w72 w98 w122 w136 w183 w196 w239 _ w279 w301]
      tunnel: [_ _ _ _ _ _ _ _ _ _ _ _ TRUE ("Priority Message? (F)") _] -> w15
      tunnel: w10 -> [_ w31 _ _ _ _ _ _ _ _ _ _ _ _]
      tunnel: w8 -> [w22 w39 w42 w66 w79 w96 w119 w137 w180 w192 w235 w261 w284 w299]
      tunnel: "Used functions" -> [_ _ _ _ _ w103 w126 w139 _ w200 w243 _ w285 _]
      tunnel: [w22 w37 w42 w66 w79 w93 w121 w138 w182 w194 w237 w261 w284 w299] -> w7
      frame Default {
        # "The Defualt Case run if there is a message that isn't defined in any of the other cases.\nOutput a program error"
        n7 = Format Into String(format string="The invalid message string \"%s\" was  received in the XYZ Stage Loop", w24) -> (resulting string=w26:string)  [unwired: 2 in, 1 out]
        n8 = call <vilib>:"Error Cluster From Error Code.vi"("error message (\"\")"=w26, "error code (0)"=5001) -> ("error out"=w23:errorcluster)  [unwired: 2 in, 5 out]
      }
      frame "Initialize" {
        n9 = Unbundle By Name(w40) -> ("XYZ Stage"=w35:refnum<queue>, "Message Handler Loop"=w32:refnum<queue>)
        n10 = call "Enqueue Message (Single).vi"("error in (no error)"=w28, "Message"="XYZ Stage - Update Refnums", "Message Queue"=w32) -> ("error out"=w34:errorcluster)  [unwired: 1 in, 7 out]
        n11 = call "Enqueue Message (Single).vi"("error in (no error)"=w34, "Message Data"=w31, "Message"="XYZ Stage - Set UI", "Message Queue"=w32) -> ("error out"=w30:errorcluster)  [unwired: 7 out]
        n12 = call "Enqueue Message (Single).vi"("error in (no error)"=w30, "Message"="Check if Refnum Update", "Message Queue"=w35) -> ("error out"=w29:errorcluster)  [unwired: 1 in, 7 out]
        n13 = Bundle By Name(cluster=w39, "Configuration"=w31) -> (w37:T58)
      }
      frame "Check if Refnum Update" {
        n14 = Unbundle By Name(w42) -> ("Initialization.Update Refnums"=w41:bool)
        n15 = case shown="False" w41 {
          tunnel: w45 -> [w50 w55]
          tunnel: [w47 w52] -> w44
          tunnel: w43 -> [w46 w51]
          frame True {
            n16 = Unbundle By Name(w50) -> ("XYZ Stage"=w48:refnum<queue>)
            n17 = call "Enqueue Message (Single).vi"("error in (no error)"=w46, "Message"="Continue Initialize", "Message Queue"=w48) -> ("error out"=w47:errorcluster)  [unwired: 1 in, 7 out]
          }
          frame False {
            n18 = Unbundle By Name(w55) -> ("XYZ Stage"=w53:refnum<queue>)
            n19 = call "Enqueue Message (Single).vi"("error in (no error)"=w51, "Message"="Check if Refnum Update", "Message Queue"=w53) -> ("error out"=w52:errorcluster)  [unwired: 1 in, 7 out]
          }
        }
      }
      frame "Continue Initialize" {
        n20 = Unbundle By Name(w58) -> ("Save Data.Ready"=w59:refnum<notifier>)
        n21 = Wait on Notification(notifier=w59, error in (no error)=w57) -> (error out=w56:errorcluster)  [unwired: 2 in, 3 out]
        n22 = Unbundle By Name(w66) -> ("Configuration.Connection Settings.Tango VISA"=w65:refnum<visa-resource-name>)
        n23 = Unbundle By Name(w71) -> ("XYZ Stage"=w62:refnum<queue>)
        n24 = call "Enqueue Message (Single).vi"("error in (no error)"=w56, "Message"="Set To Default", "Message Queue"=w62) -> ("error out"=w63:errorcluster)  [unwired: 1 in, 7 out]
        n25 = call "Enqueue Message (Single).vi"("error in (no error)"=w63, "Message Data"=w65, "Message"="Update Visa Session", "Message Queue"=w62) -> ("error out"=w61:errorcluster)  [unwired: 7 out]
        n26 = call "Enqueue Message (Single).vi"("error in (no error)"=w61, "Message"="Get Status", "Message Queue"=w62) -> ("error out"=w69:errorcluster)  [unwired: 1 in, 7 out]
        n27 = call "Enqueue Message (Single).vi"("error in (no error)"=w69, "Message"="Ready", "Message Queue"=w62) -> ("error out"=w68:errorcluster)  [unwired: 1 in, 7 out]
      }
      frame "Ready" {
        n28 = Unbundle By Name(w79) -> ("Initialization.Update Visa Session"=w80:bool, "Initialization.Set To Default"=w76:bool, "Initialization.Get Status"=w77:bool, "Initialization.Update Refnums"=w78:bool)
        n29 = Compound Arithmetic op=AND(w80, w76, w77, w78) -> (w81:bool)
        n30 = case shown="True" w81 {
          tunnel: [w84 w89] -> w73
          tunnel: w75 -> [w83 w88]
          tunnel: w74 -> [w82 _]
          tunnel: w72 -> [_ w87]
          frame False {
            n31 = Unbundle By Name(w82) -> ("XYZ Stage"=w86:refnum<queue>)
            n32 = call "Enqueue Message (Single).vi"("error in (no error)"=w83, "Message"="Ready", "Message Queue"=w86) -> ("error out"=w84:errorcluster)  [unwired: 1 in, 7 out]
          }
          frame True {
            n33 = Unbundle By Name(w87) -> ("XYZ Stage.Ready"=w90:refnum<notifier>)
            n34 = Send Notification(notification=TRUE, notifier=w90, error in (no error)=w88) -> (error out=w89:errorcluster)  [unwired: 1 out]
          }
        }
      }
      frame "Update Visa Session" {
        n35 = Unbundle By Name(w96) -> ("Configuration.Connection Settings.Tango VISA"=w95:refnum<visa-resource-name>)
        n36 = Variant To Data(error in=w104, type=w95, Variant=w106) -> (data=w94:refnum<visa-resource-name>, error out=w105:errorcluster)
        n37 = Bundle By Name(cluster=w96, "Initialization.Update Visa Session"=TRUE, "Configuration.Connection Settings.Tango VISA"=w94) -> (w93:T58)
        n38 = Unbundle By Name(w93) -> ("Configuration.Connection Settings"=w92:T25)
        n39 = case shown="True" w103 {
          tunnel: w105 -> [w110 w115]
          tunnel: [w109 w113] -> w99
          tunnel: w98 -> [w112 _]
          tunnel: w92 -> [_ w114]
          frame False {
            n40 = Unbundle By Name(w112) -> ("XYZ Stage.Status"=w111:refnum<notifier>)
            n41 = One Button Dialog(message="XYZ Stage VISA Session Updated" ("button name (\"OK\")")) -> ()  [unwired: 2 out]
            n42 = Send Notification(notification="Connected", notifier=w111, error in (no error)=w110) -> (error out=w109:errorcluster)  [unwired: 1 out]
          }
          frame True {
            n43 = call "XYZ.vi"("Function"=XYZ_Function."Connect", "Connection Settings"=w114, "Error In (no error)"=w115) -> ("Error Out"=w113:errorcluster)  [unwired: 10 in, 2 out]
          }
        }
        n44 = call "Update Status.vi"("error in"=w99, "String"="XYZ Stage VISA Session Updated" ("button name (\"OK\")"), "Message Queues out"=w101) -> ("error out"=w102:errorcluster)  [unwired: 8 out]
      }
      frame "Set To Default" {
        w117 = "XYZ Stage Set To Default" ("button name (\"OK\")")
        n45 = case shown="True" w126 {
          tunnel: w118 -> [w128 w130]
          tunnel: [w128 w129] -> w123
          tunnel: w122 -> [_ _]
          tunnel: w117 -> [w127 _]
          frame False {
            n46 = One Button Dialog(message=w127) -> ()  [unwired: 2 out]
          }
          frame True {
            n47 = call "XYZ.vi"("Function"=XYZ_Function."Initialize", "Error In (no error)"=w130) -> ("Error Out"=w129:errorcluster)  [unwired: 11 in, 2 out]
          }
        }
        n48 = Bundle By Name(cluster=w119, "Initialization.Set To Default"=TRUE ("Initialization.Update Visa Session")) -> (w121:T58)
        n49 = call "Update Status.vi"("error in"=w123, "String"=w117, "Message Queues out"=w124) -> ("error out"=w125:errorcluster)  [unwired: 8 out]
      }
      frame "Get Status" {
        n50 = Unbundle By Name(w137) -> ("Initialization.Update Refnums"=w133:bool)
        n51 = case shown="True" w133 {
          tunnel: w139 -> [_ w154]
          tunnel: [w140 w153] -> w138
          tunnel: w137 -> [w140 w152]
          tunnel: [w141 w147] -> w132
          tunnel: w136 -> [_ w151]
          tunnel: w135 -> [w143 w149]
          tunnel: w134 -> [w142 w150]
          frame False {
            n52 = Unbundle By Name(w143) -> ("XYZ Stage"=w145:refnum<queue>)
            n53 = call "Enqueue Message (Single).vi"("error in (no error)"=w142, "Message"="Get Status", "Message Queue"=w145) -> ("error out"=w141:errorcluster)  [unwired: 1 in, 7 out]
          }
          frame True {
            n54 = case shown="True" w154 {
              tunnel: w150 -> [w157 w169]
              tunnel: [w156 w168] -> w148
              tunnel: w152 -> [w165 w173]
              tunnel: [w164 w171] -> w153
              tunnel: w151 -> [w159 _]
              tunnel: [w158 w167] -> w146
              frame False {
                w158 = "XYZ Stage Status Updated" ("button name (\"OK\")")
                n55 = Bundle By Name(cluster=w165, "Initialization.Get Status"=TRUE ("Initialization.Configure Integration Time")) -> (w164:T58)
                n56 = Unbundle By Name(w159) -> ("XYZ Stage.Status"=w162:refnum<notifier>)
                n57 = call "Dialog.vi"("error in (no error)"=w157, "message"=w158) -> ("error out"=w155:errorcluster)  [unwired: 1 in, 8 out]
                n58 = Send Notification(notification="Status Acquired", notifier=w162, error in (no error)=w157) -> (error out=w160:errorcluster)  [unwired: 1 out]
                n59 = Merge Errors(w155, w160) -> (w156:errorcluster)
              }
              frame True {
                n60 = call "XYZ.vi"("Function"=XYZ_Function."Get Status", "Error In (no error)"=w169) -> ("Status"=w166:T62, "Error Out"=w168:errorcluster)  [unwired: 11 in, 1 out]
                n61 = Bundle By Name(cluster=w173, "Initialization.Get Status"=TRUE ("Initialization.Configure Integration Time")) -> (w171:T58)
                n62 = call "XYZ Position to String.vi"("Status"=w166) -> ("String"=w167:string)
              }
            }
            n63 = call "Update Status.vi"("error in"=w148, "String"=w146, "Message Queues out"=w149) -> ("error out"=w147:errorcluster)  [unwired: 8 out]
          }
        }
      }
      frame "Update Refnums" {
        n64 = Unbundle By Name(w180) -> ("Refnums"=w179:T59)
        n65 = Variant To Data(error in=w187, type=w179, Variant=w188) -> (data=w174:T59, error out=w175:errorcluster)
        n66 = Unbundle By Name(w183) -> ("XYZ Stage"=w177:T52)
        n67 = Bundle By Name(cluster=w180, "Initialization.Update Refnums"=TRUE, "Refnums"=w174) -> (w182:T58)
        n68 = call "XYZ.vi"("Function"=XYZ_Function."Update Refnums", "Notifications"=w177, "Refnums"=w174, "Error In (no error)"=w175) -> ("Error Out"=w176:errorcluster)  [unwired: 9 in, 2 out]
        n69 = call "Update Status.vi"("error in"=w176, "String"="XYZ Stage Refnums Updated" ("button name (\"OK\")"), "Message Queues out"=w184) -> ("error out"=w186:errorcluster)  [unwired: 8 out]
      }
      frame "Move" {
        n70 = Unbundle By Name(w192) -> ("Configuration"=w198:T24)
        n71 = Variant To Data(error in=w201, type=w198, Variant=w203) -> (data=w193:T24, error out=w202:errorcluster)
        n72 = Unbundle By Name(w193) -> ("Coordinate Control"=w190:T27)
        n73 = Bundle By Name(cluster=w192, "Configuration.Coordinate Control"=w190) -> (w191:T58)
        n74 = call "XYZ Coordinate to String.vi"("Coordinate Control"=w190) -> ("String"=w189:string)
        n75 = case shown="True" w200 {
          tunnel: w202 -> [w206 w216]
          tunnel: [w205 w215] -> w197
          tunnel: w196 -> [w210 _]
          tunnel: w189 -> [w209 _]
          tunnel: w191 -> [w207 w214]
          tunnel: [w207 w214] -> w194
          tunnel: w190 -> [_ w213]
          frame False {
            n76 = Unbundle By Name(w210) -> ("XYZ Stage.Status"=w212:refnum<notifier>)
            n77 = Send Notification(notification="Motion Done" ("button name (\"OK\")"), notifier=w212, error in (no error)=w206) -> (error out=w211:errorcluster)  [unwired: 1 out]
            n78 = call "Dialog.vi"("error in (no error)"=w206, "message"=w209) -> ("error out"=w204:errorcluster)  [unwired: 1 in, 8 out]
            n79 = Merge Errors(w211, w204) -> (w205:errorcluster)
          }
          frame True {
            n80 = call "XYZ.vi"("Function"=XYZ_Function."Move with Backlash Compensation", "Coordinate Control"=w213, "Error In (no error)"=w216) -> ("Error Out"=w215:errorcluster)  [unwired: 10 in, 2 out]
          }
        }
        n81 = call "Update Status.vi"("error in"=w197, "String"=w189, "Message Queues out"=w195) -> ("error out"=w199:errorcluster)  [unwired: 8 out]
      }
      frame "Manual Control" {
        n82 = Unbundle By Name(w235) -> ("Configuration"=w241:T24)
        n83 = Variant To Data(error in=w244, type=w241, Variant=w246) -> (data=w236:T24, error out=w245:errorcluster)
        n84 = Unbundle By Name(w236) -> ("Manual Control"=w221:T26)
        n85 = Bundle By Name(cluster=w235, "Configuration.Manual Control"=w221) -> (w234:T58)
        n86 = Unbundle By Name(w221) -> ("North"=w232:bool, "South"=w231:bool, "West"=w226:bool, "East"=w225:bool, "Down"=w230:bool, "Up"=w229:bool, "XY Step"=w228:dbl, "Z step"=w227:dbl)
        n87 = call "XYZ Step.vi"("Step Size"=w228, "Negative"=w231, "Positive"=w232) -> ("Relative Movement"=w223:dbl)
        n88 = call "XYZ Step.vi"("Step Size"=w228, "Negative"=w225, "Positive"=w226) -> ("Relative Movement"=w224:dbl)
        n89 = call "XYZ Step.vi"("Step Size"=w227, "Negative"=w229, "Positive"=w230) -> ("Relative Movement"=w222:dbl)
        n90 = Build Array(w224, w223, w222) -> (w218:dbl[])
        n91 = Bundle By Name(cluster=T27 {"Motion Mode"=enum."Relative", "Destination [mm]"=[]} ("Coordinate Control"), "Destination [mm]"=w218) -> (w219:T27)
        n92 = call "XYZ Coordinate to String.vi"("Coordinate Control"=w219) -> ("String"=w233:string)
        n93 = case shown="True" w243 {
          tunnel: w245 -> [w249 w259]
          tunnel: [w248 w258] -> w240
          tunnel: w239 -> [w253 _]
          tunnel: w233 -> [w252 _]
          tunnel: w234 -> [w250 w257]
          tunnel: [w250 w257] -> w237
          tunnel: w221 -> [_ w256]
          frame False {
            n94 = Unbundle By Name(w253) -> ("XYZ Stage.Status"=w255:refnum<notifier>)
            n95 = Send Notification(notification="Motion Done" ("button name (\"OK\")"), notifier=w255, error in (no error)=w249) -> (error out=w254:errorcluster)  [unwired: 1 out]
            n96 = call "Dialog.vi"("error in (no error)"=w249, "message"=w252) -> ("error out"=w247:errorcluster)  [unwired: 1 in, 8 out]
            n97 = Merge Errors(w254, w247) -> (w248:errorcluster)
          }
          frame True {
            n98 = call "XYZ.vi"("Function"=XYZ_Function."Manual Control", "Manual Control"=w256, "Error In (no error)"=w259) -> ("Error Out"=w258:errorcluster)  [unwired: 10 in, 2 out]
          }
        }
        n99 = call "Update Status.vi"("error in"=w240, "String"=w233, "Message Queues out"=w238) -> ("error out"=w242:errorcluster)  [unwired: 8 out]
      }
      frame "Error" {
        # "Clear Errors to avoid getting stuck \nin repeating this case"
        # "Add here Cases that are handled \nalready by the Message Handler Loop"
        n100 = Variant To Data(error in=w269, type=errorcluster {"status"=FALSE, "code"=0, "source"=""} ("error out"), Variant=w262) -> (data=w268:errorcluster, error out=w267:errorcluster)
        n101 = Merge Errors(w268, w267) -> (w266:errorcluster)
        n102 = Unbundle By Name(w270) -> ("Message Handler Loop"=w272:refnum<queue>)
        n103 = Unbundle By Name(w266) -> ("code"=w263:i32)
        n104 = case shown="Default" w263 {
          tunnel: w272 -> [w276]
          tunnel: w266 -> [w274]
          tunnel: [w273] -> w265
          frame Default {
            n105 = call "Enqueue Message (Single).vi"("Message Data"=w274, "Message"="Error", "Message Queue"=w276) -> ("error out"=w273:errorcluster)  [unwired: 1 in, 7 out]
          }
        }
        n106 = call <vilib>:"Clear Errors.vi"("error in (no error)"=w265) -> ("error out"=w264:errorcluster)  [unwired: 1 in, 5 out]
      }
      frame "Exit" {
        w282 = TRUE ("Priority Message? (F)")
        # "Stop the VI"
        n107 = case shown="True" w285 {
          tunnel: w287 -> [w293 w298]
          tunnel: [w292 w297] -> w286
          tunnel: w279 -> [w291 _]
          frame False {
            n108 = Unbundle By Name(w291) -> ("XYZ Stage.Status"=w294:refnum<notifier>)
            n109 = Send Notification(notification="Disconnected", notifier=w294, error in (no error)=w293) -> (error out=w292:errorcluster)  [unwired: 1 out]
          }
          frame True {
            n110 = call "XYZ.vi"("Function"=XYZ_Function."Disconnect", "Error In (no error)"=w298) -> ("Error Out"=w297:errorcluster)  [unwired: 11 in, 2 out]
          }
        }
        n111 = Unbundle By Name(w289) -> ("XYZ Stage"=w290:refnum<queue>)
        n112 = Release Queue(queue=w290, error in (no error)=w286) -> (error out=w278:errorcluster)  [unwired: 3 out]
        n113 = Unbundle By Name(w279) -> ("XYZ Stage.Exit"=w283:refnum<notifier>, "XYZ Stage.Ready"=w280:refnum<notifier>)
        n114 = Send Notification(notification=w282, notifier=w280, error in (no error)=w278) -> (error out=w281:errorcluster)  [unwired: 1 out]
        n115 = Send Notification(notification=w282, notifier=w283, error in (no error)=w281) -> (error out=w277:errorcluster)  [unwired: 1 out]
      }
      frame "Notify Status" {
        n116 = Unbundle By Name(w301) -> ("XYZ Stage.Instrument Data"=w300:refnum<notifier>)
        n117 = Send Notification(notification=w299, notifier=w300, error in (no error)=w303) -> (error out=w302:errorcluster)  [unwired: 1 out]
      }
    }
    n118 = call "Message Handling Loop.vi"("error in (no error)"=w14, "Message Queue"=w12) -> ("dup error in"=w13:errorcluster)  [unwired: 9 out]
  }
  "error out" <- w2
